vi "AM Get Mean Data.vi"(11 "Array":dbl[](array[numeric])) -> (3 "Data":dbl[](array[numeric]))   [LabVIEW 2020, in "Test Driver.lvlib"]
uses:
  Test Driver.lvlib
  <vilib>/Analysis/baseanly.llb/Mean (DBL).vi
  <vilib>/Analysis/NI_AALBase.lvlib
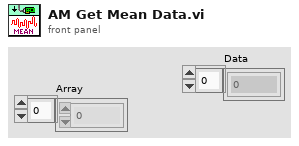
[diagram p1: front panel]
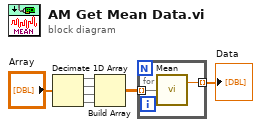
[diagram p0: block diagram]
diagram:
  n1 = Decimate 1D Array("Array") -> (w3:dbl[], w4:dbl[], w5:dbl[], w6:dbl[])
  n2 = Build Array(w3, w4, w5, w6) -> (w7:dbl[][])
  n3 = for {
    tunnel: w7 -> [w9] mode=indexing
    tunnel: [w8] -> w1 mode=indexing
    n4 = call-poly <vilib>:"Mean.vi"("X"=w9) -> ("mean"=w8:dbl)  [unwired: 1 out]
  }
  "Data" <- w1
